vi "OpenVI.vi"(0 "#":i32, 2 "Slides":T1[](array[typedef]), 3 "Scene.Object in":refnum<vi>, 4 "reference":refnum<vi>) -> (1 "New #":i32, 5 "Scene.Object Out":refnum<vi>)   [LabVIEW 2010]
uses:
  SlideTypeDef.ctl
  LVPresent_Globals.vi
panel:
  out "queue":string
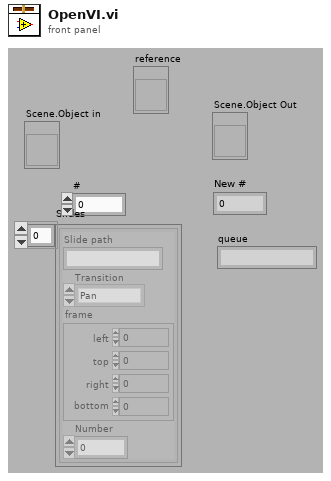
[diagram p1: front panel]
types:
  T1 = typedef "SlideTypeDef.ctl" = cluster{"Slide path":string, "Transition":enum16{"Pan", "Zoom-pan-zoom", "Zoom-wait-Zoom"}, "frame":cluster{"left":i16, "top":i16, "right":i16, "bottom":i16}, "Number":i32}
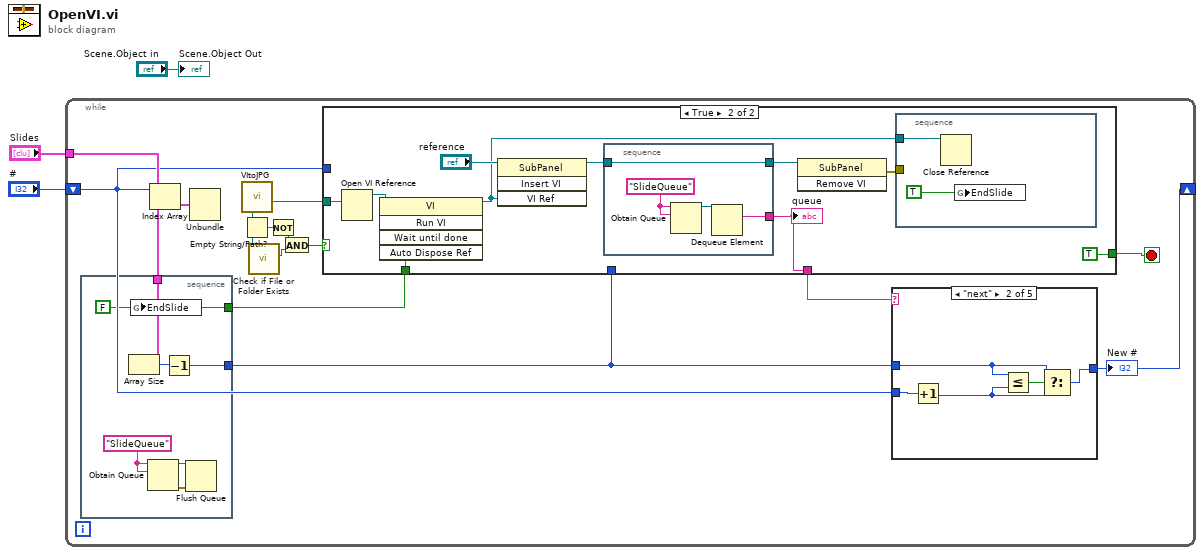
[diagram p0: block diagram]
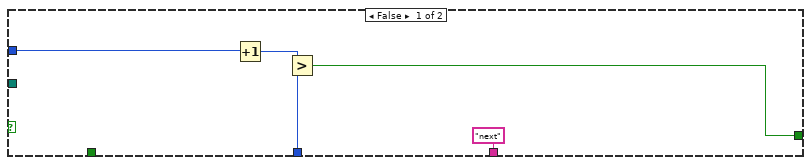
[diagram p2: hidden frame]
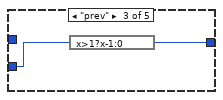
[diagram p4: hidden frame]
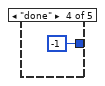
[diagram p5: hidden frame]
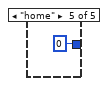
[diagram p6: hidden frame]
diagram:
  n1 = while {
    tunnel: "Slides" -> [w13]
    shift-right: [w12] -> _
    shift-left: "#" -> [w10]
    stop <- w11 stop-if-true
    n2 = stacked-sequence {
      tunnel: [w48] -> w16
      tunnel: w13 -> [w50]
      tunnel: [w49] -> w9
      frame #0 {
        w54 = "SlideQueue" ("name (unnamed)")
        w48 = FALSE ("Front Panel Window:Open")
        n3 = Array Size(array=w50) -> (size(s)=w51:i32)
        n4 = global write "LVPresent_Globals.vi" "EndSlide"(w48) -> ()
        n5 = Obtain Queue(name (unnamed)=w54, element data type=w54) -> (queue out=w53:refnum<queue>, error out=w52:errorcluster)  [unwired: 3 in, 1 out]
        n6 = Decrement(x=w51) -> (x-1=w49:i32)
        n7 = Flush Queue(queue=w53, error in (no error)=w52) -> ()  [unwired: 3 out]
      }
    }
    n8 = Index Array(array=w13, index=w10) -> (element=w15:T1)
    n9 = Unbundle(w15) -> ()  [unwired: 4 out]
    n10 = call "VItoJPG.vi"() -> ("appended path"=w8:path)  [unwired: 2 in]
    n11 = Empty String/Path?(string/path=w8) -> (empty?=w7:bool)
    n12 = call <vilib>:"Check if File or Folder Exists.vi"("path"=w8) -> ("file or folder exists?"=w6:bool)  [unwired: 8 in, 2 out]
    n13 = Not(x=w7) -> (.not. x?=w5:bool)
    n14 = And(x=w5, y=w6) -> (x .and. y?=w4:bool)
    n15 = case shown="True" w4 {
      tunnel: w16 -> [_ w29]
      tunnel: ["next" ("name (unnamed)") w26] -> w14
      tunnel: w8 -> [_ w23]
      tunnel: [w17 TRUE] -> w11
      tunnel: w10 -> [w20 _]
      tunnel: w9 -> [w18 _]
      frame False {
        n16 = Increment(x=w20) -> (x+1=w19:i32)
        n17 = Greater?(x=w19, y=w18) -> (0:w17:bool)
      }
      frame True {
        n18 = Open VI Reference(vi path=w23) -> (vi reference=w25:refnum<vi>)  [unwired: 5 in, 1 out]
        n19 = invoke class="VI" method="Run VI"(reference=w25, "Wait until done"=w29, "Auto Dispose Ref"=w29) -> (reference out=w24:refnum<vi>)  [unwired: 2 in, 4 out]
        n20 = invoke on="Invoke Node" class="SubPanel" method="Insert VI"(reference="reference", "VI Ref"=w24) -> (reference out=w27:refnum<vi>)  [unwired: 2 in, 3 out]
        n21 = stacked-sequence {
          tunnel: [w37] -> w26
          tunnel: [w34] -> w28
          tunnel: w27 -> [w34]
          frame #0 {
            w36 = "SlideQueue" ("name (unnamed)")
            n22 = Obtain Queue(name (unnamed)=w36, element data type=w36) -> (queue out=w35:refnum<queue>)  [unwired: 3 in, 2 out]
            n23 = Dequeue Element(queue=w35) -> (element=w37:string)  [unwired: 2 in, 3 out]
          }
        }
        "queue" <- w26
        n24 = invoke on="Invoke Node" class="SubPanel" method="Remove VI"(reference=w28) -> (error out=w30:errorcluster)  [unwired: 2 in, 2 out]
        n25 = stacked-sequence {
          tunnel: w30 -> [_]
          tunnel: w24 -> [w32]
          frame #0 {
            n26 = Close Reference(reference=w32) -> ()  [unwired: 1 in, 1 out]
            n27 = global write "LVPresent_Globals.vi" "EndSlide"(TRUE) -> ()
          }
        }
      }
    }
    n28 = case shown="\"next\"" w14 {
      tunnel: [w38 w41 w44 -1 ("Resolution") 0 ("Resolution")] -> w12
      tunnel: w10 -> [w38 w43 w45 _ _]
      tunnel: w9 -> [_ w39 _ _ _]
      frame Default {
      }
      frame "next" {
        n29 = Increment(x=w43) -> (x+1=w40:i32)
        n30 = Less Or Equal?(x=w39, y=w40) -> (x <= y?=w42:bool)
        n31 = Select(t=w39, s=w42, f=w40) -> (s? t:f=w41:i32)
      }
      frame "prev" {
        n32 = expression code="x>1?x-1:0"(w45) -> (w44:i32)
      }
      frame "done" {
      }
      frame "home" {
      }
    }
    "New #" <- w12
  }
  "Scene.Object Out" <- "Scene.Object in"
